vi "Write Control Index.vi"(8 "error in (no error)":errorcluster, 10 "Control Index":i32, 11 "UI-Bus_Boolean in":refnum<class "UI-Bus_I16.lvclass">) -> (0 "error out":errorcluster, 3 "UI-Bus_Boolean out":refnum<class "UI-Bus_I16.lvclass">)   [LabVIEW 2021, in "UI-Bus_I16.lvclass"]
uses:
  UI-Bus_I16.lvclass
  UI-Bus_I16.lvclass/UI-Bus_I16.ctl
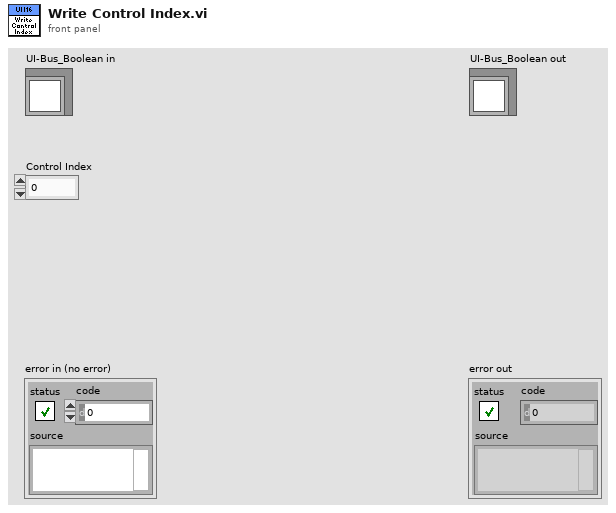
[diagram p1: front panel]
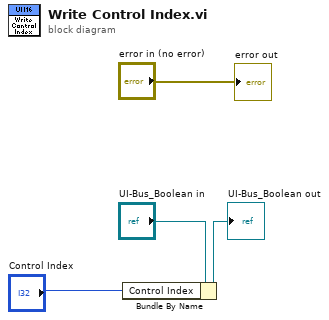
[diagram p0: block diagram]
diagram:
  n1 = Bundle By Name(cluster="UI-Bus_Boolean in", "Control Index"="Control Index") -> (→"UI-Bus_Boolean out":refnum<class "UI-Bus_I16.lvclass">)
  "error out" <- "error in (no error)"
